vi "test_Add Response WaitSec.vi"(8 "error in (no error)":errorcluster, 11 "TestCase in":refnum<class "Instrument Addon Scripting API Messages Unit Tests.lvclass">) -> (0 "error out":errorcluster, 3 "TestCase out":refnum<class "Instrument Addon Scripting API Messages Unit Tests.lvclass">)   [LabVIEW 2018, in "Instrument Addon Scripting API Messages Unit Tests.lvclass"]
uses:
  Instrument Addon Scripting API Messages Unit Tests.lvclass
  Addon/Addon Shared/Types/FG Control.ctl
  APIs/Scripting API/TypeDefs/Wait Response Settings.ctl
  APIs/Scripting API/TypeDefs/Linked Channel.ctl
  <vilib>/NI Veristand/Custom Device API/Custom Device Item Ref.ctl
  Addon/Addon Shared/Types/Response Parameters.ctl
  Addon/Addon Shared/Types/Linked Channel Cluster.ctl
  Addon/Addon Shared/Types/Response Wait Type.ctl
  Addon/Addon Shared/SubVIs/Constants.vi
  <vilib>/NI/NI VeriStand Advanced SysDef API/_SubVIs/SysDef.Search.GUID.vi
  <vilib>/NI Veristand/Custom Device API/NI VeriStand - Get Item Property.vi
  <vilib>/NI Veristand/Custom Device API/Get Item Property (String).vi
  <vilib>/NI Veristand/Custom Device API/Get Item Property (String Array).vi
  <vilib>/NI Veristand/Custom Device API/Get Item Property (Double).vi
  <vilib>/NI Veristand/Custom Device API/Get Item Property (U32).vi
  <vilib>/NI Veristand/Custom Device API/Get Item Property (Boolean).vi
  <vilib>/NI Veristand/Custom Device API/NI VeriStand - Set Item Property.vi
  <vilib>/NI Veristand/Custom Device API/Set Item Property (String).vi
  <vilib>/NI Veristand/Custom Device API/Set Item Property (String Array).vi
  <vilib>/NI Veristand/Custom Device API/Set Item Property (Double).vi
  <vilib>/NI Veristand/Custom Device API/Set Item Property (U32).vi
  <vilib>/NI Veristand/Custom Device API/Set Item Property (Boolean).vi
  APIs/Scripting API/Messages/Add Response - Wait (sec).vi
  <vilib>/addons/_JKI Toolkits/VI Tester/TestCase.llb/TestCase.lvclass
  Instrument Addon Scripting API Test Assets/Instrument Addon Scripting API Test Assets.lvclass
  APIs/Scripting API/Instrument Addon Scripting API.lvlib
  <vilib>/NI Veristand/Custom Device API/Custom Device API.lvlib
  Addon/Addon Shared/Instrument Addon Shared.lvlib
  <vilib>/NI/NI VeriStand Advanced SysDef API/SysDef API/Advanced System Definition.lvlib
  C:/Program Files (x86)/National Instruments/LabVIEW 2018/vi.lib/addons/_JKI Toolkits/VI Tester/TestCase.llb/TestCase.lvclass
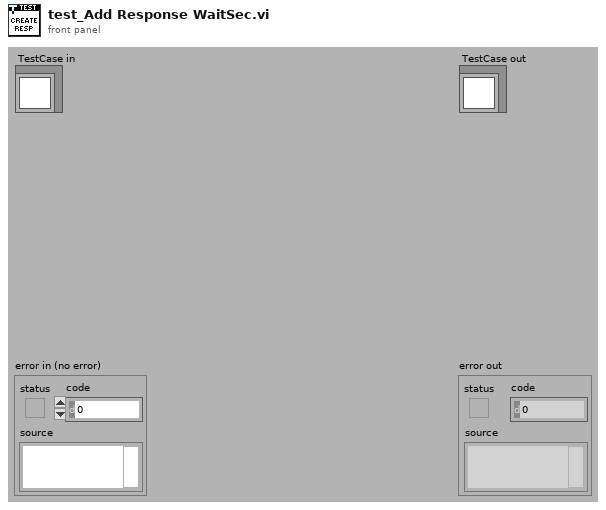
[diagram p1: front panel]
types:
  T1 = typedef "Instrument Addon Scripting API.lvlib/Wait Response Settings.ctl" = cluster{"Response Format":string, "Linked Channels":T2[], "Wait value (sec)":dbl, "Use Wait Channel":bool, "Channel Refnum":T3}
  T2 = typedef "Instrument Addon Scripting API.lvlib/Linked Channel.ctl" = cluster{"Variable Name":string, "Channel Refnum":T3}
  T3 = typedef "Custom Device API.lvlib/Custom Device Item Ref.ctl" = u64
  T4 = typedef "Instrument Addon Shared.lvlib/FG Control.ctl" = enum16{"Get", "Set"}
  T5 = typedef "Instrument Addon Shared.lvlib/Response Parameters.ctl" = cluster{"Response":string, "Linked Channels":T6[], "Type Value":dbl, "Wait Type":T7, "Use Channel":bool, "Channel Path":string}
  T6 = typedef "Instrument Addon Shared.lvlib/Linked Channel Cluster.ctl" = cluster{"Variable Name":string, "GUID":string}
  T7 = typedef "Instrument Addon Shared.lvlib/Response Wait Type.ctl" = enum16{"Byte Count", "Wait sec"}
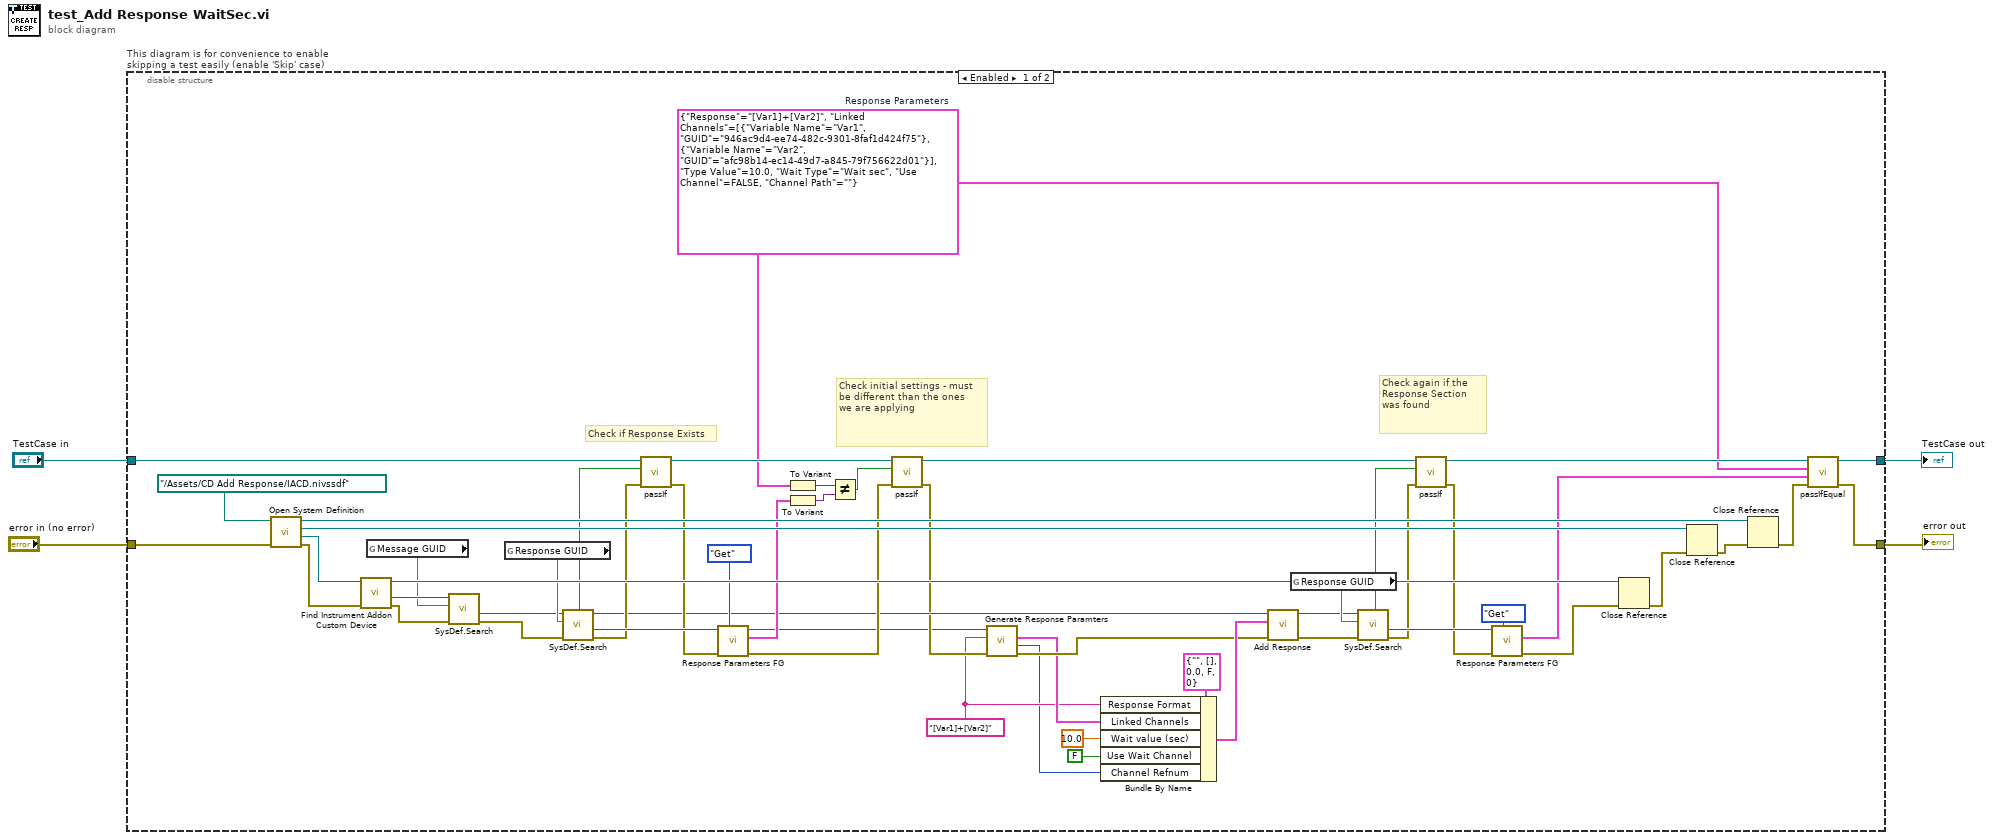
[diagram p0: block diagram]
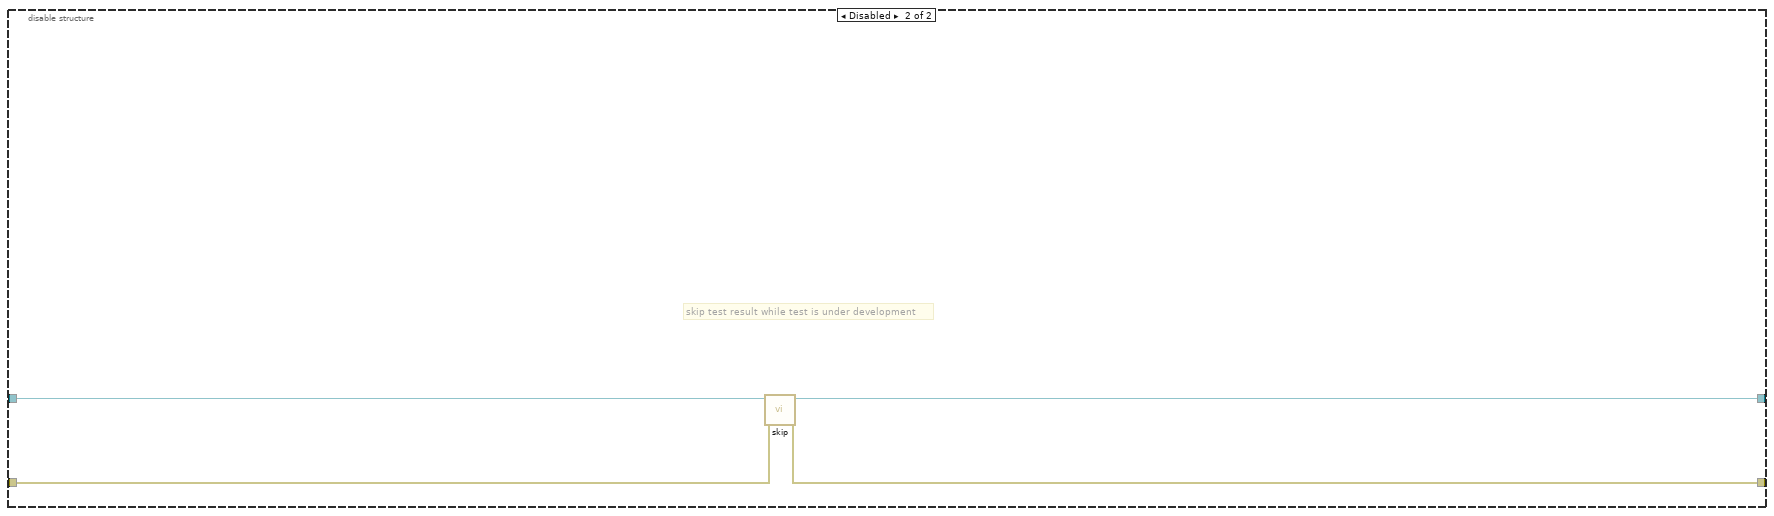
[diagram p2: hidden frame]
diagram:
  n1 = disable-structure "This diagram is for convenience to enable skipping a test easily (enable 'Skip' case)" shown="Enabled" {
    disable-tunnel: "TestCase in" -> [w32 w62]
    disable-tunnel: [w41 w60] -> w1
    disable-tunnel: [w40 w61] -> w3
    disable-tunnel: "error in (no error)" -> [w57 w59]
    frame Enabled {
      w11 = T5 {"Response"="[Var1]+[Var2]", "Linked Channels"=[{"Variable Name"="Var1", "GUID"="946ac9d4-ee74-482c-9301-8faf1d424f75"}, {"Variable Name"="Var2", "GUID"="afc98b14-ec14-49d7-a845-79f756622d01"}], "Type Value"=10.0, "Wait Type"=enum."Wait sec", "Use Channel"=FALSE, "Channel Path"=""}  # Response Parameters
      w6 = "[Var1]+[Var2]" ("Response Format")
      # "Check again if the Response Section was found"
      # "Check initial settings - must be different than the ones\nwe are applying"
      # "Check if Response Exists"
      n2 = call "Open System Definition.vi"("error in (no error)"=w57, "System Definition File"=path "../Assets/CD Add Response/IACD.nivssdf" ("SDF file")) -> ("error out"=w55:errorcluster, "Target Refnum"=w54:refnum<k24>, "Root Refnum"=w53:refnum<k24>, "System Definition Refnum"=w44:refnum<k24>)  [unwired: 6 in]
      n3 = call "Find Instrument Addon Custom Device.vi"("error in"=w55, "target in"=w54) -> ("error out"=w15:errorcluster, "NodeID"=w16:u64, "target out"=w52:refnum<k24>)  [unwired: 7 in]
      n4 = global read "Constants.vi" "Message GUID"() -> (w14:string)
      n5 = call-poly <vilib>:"SysDef.Search.vi"("error in (no error)"=w15, "GUID"=w14, "nodeID"=w16) -> ("error out"=w13:errorcluster, "Value out"=w12:u64)  [unwired: 5 in, 2 out]
      n6 = global read "Constants.vi" "Response GUID"() -> (w37:string)
      n7 = call-poly <vilib>:"SysDef.Search.vi"("error in (no error)"=w13, "GUID"=w37, "nodeID"=w12) -> ("error out"=w30:errorcluster, "Value out"=w38:u64, "nodeID out"=w17:u64, "Found?"=w31:bool)  [unwired: 5 in]
      n8 = call-dynamic "passIf.vi"("error in (no error)"=w30, "pass"=w31, "TestCase in"=w32) -> ("error out"=w29:errorcluster, "TestCase out"=w28:refnum<class "Instrument Addon Scripting API Messages Unit Tests.lvclass">)  [unwired: 7 in]
      n9 = call "Response Parameters FG.vi"("Action"=FG_Control."Get", "error in (no error)"=w29, "Item Ref in"=w38) -> ("error out"=w27:errorcluster, "Response Parameters"=w36:T5, "Item Ref out"=w8:T3)  [unwired: 6 in]
      n10 = To Variant(anything=w11) -> (Variant=w35:variant)
      n11 = To Variant(anything=w36) -> (Variant=w34:variant)
      n12 = Not Equal?(x=w35, y=w34) -> (x != y?=w33:bool)
      n13 = call-dynamic "passIf.vi"("error in (no error)"=w27, "pass"=w33, "TestCase in"=w28) -> ("error out"=w10:errorcluster, "TestCase out"=w26:refnum<class "Instrument Addon Scripting API Messages Unit Tests.lvclass">)  [unwired: 7 in]
      n14 = call "Generate Response Paramters.vi"("Error In"=w10, "Response String"=w6, "Response Channel in"=w8) -> ("Error Out"=w9:errorcluster, "Wait Channel Ref out"=w5:T3, "Linked Channels"=w7:T2[])  [unwired: 5 in, 1 out]
      n15 = Bundle By Name(cluster=T1 {"Response Format"="", "Linked Channels"=[], "Wait value (sec)"=0.0, "Use Wait Channel"=FALSE, "Channel Refnum"=0} ("Settings"), "Response Format"=w6, "Linked Channels"=w7, "Wait value (sec)"=10.0, "Use Wait Channel"=FALSE ("Use Byte Count channel"), "Channel Refnum"=w5) -> (w19:T1)
      n16 = call-poly "Add Response.vi"("error in (no error)"=w9, "Settings"=w19, "Message in"=w17) -> ("error out"=w47:errorcluster, "Message out"=w46:T3)  [unwired: 7 in]
      n17 = global read "Constants.vi" "Response GUID"() -> (w48:string)
      n18 = call-poly <vilib>:"SysDef.Search.vi"("error in (no error)"=w47, "GUID"=w48, "nodeID"=w46) -> ("error out"=w25:errorcluster, "Value out"=w45:u64, "Found?"=w24:bool)  [unwired: 5 in, 1 out]
      n19 = call-dynamic "passIf.vi"("error in (no error)"=w25, "pass"=w24, "TestCase in"=w26) -> ("error out"=w23:errorcluster, "TestCase out"=w22:refnum<class "Instrument Addon Scripting API Messages Unit Tests.lvclass">)  [unwired: 7 in]
      n20 = call "Response Parameters FG.vi"("Action"=FG_Control."Get", "error in (no error)"=w23, "Item Ref in"=w45) -> ("error out"=w49:errorcluster, "Response Parameters"=w18:T5)  [unwired: 6 in, 1 out]
      n21 = Close Reference(reference=w52, error in (no error)=w49) -> (error out=w56:errorcluster)
      n22 = Close Reference(reference=w53, error in (no error)=w56) -> (error out=w43:errorcluster)
      n23 = Close Reference(reference=w44, error in (no error)=w43) -> (error out=w42:errorcluster)
      n24 = call-dynamic "passIfEqual.vi"("error in (no error)"=w42, "y"=w18, "x"=w11, "TestCase in"=w22) -> ("error out"=w40:errorcluster, "TestCase out"=w41:refnum<class "Instrument Addon Scripting API Messages Unit Tests.lvclass">)  [unwired: 6 in]
    }
    frame Disabled {
      # "skip test result while test is under development"
      n25 = call <vilib>:"skip.vi"("error in (no error)"=w59, "TestCase in"=w62) -> ("error out"=w61:errorcluster, "TestCase out"=w60:refnum<class "Instrument Addon Scripting API Messages Unit Tests.lvclass">)  [unwired: 8 in]
    }
  }
  "error out" <- w3
  "TestCase out" <- w1
